vi "Build Waveform.vi"(6 "sampling config":cluster{"Fs":dbl, "#s":dbl}={"Fs"=1000.0, "#s"=1000.0} {"Fs" format="%.2p"}, 8 "error in (no error)":errorcluster, 11 "Config":T1={"Frequency"=10.0, "Voltage (V)"=1.0, "Signal type"=enum."Sine Wave", "Square wave duty cycle (%)"=50.0, "Offset (V)"=0.01, "DC shift"=FALSE} {"Square wave duty cycle (%)" format="%0.2f"}) -> (0 "error out":errorcluster, 3 "Waveform":waveform(dbl)(graph))   [LabVIEW 2019]
doc: "This example demonstrates how to acquire a continuous amount of data (Waveform) using the DAQ device's internal clock. It also shows how to synchronize two devices for different device families (E Series, S Series, M Series, X Series, DSA, and SC Express), to simultaneously acquire the data.\n\nFor instructions on how to connect your signals to the DAQ device, refer to your device documentation."
uses:
  <vilib>/measure/NI_MABase.lvlib
panel:
  # "Generate Waveform"
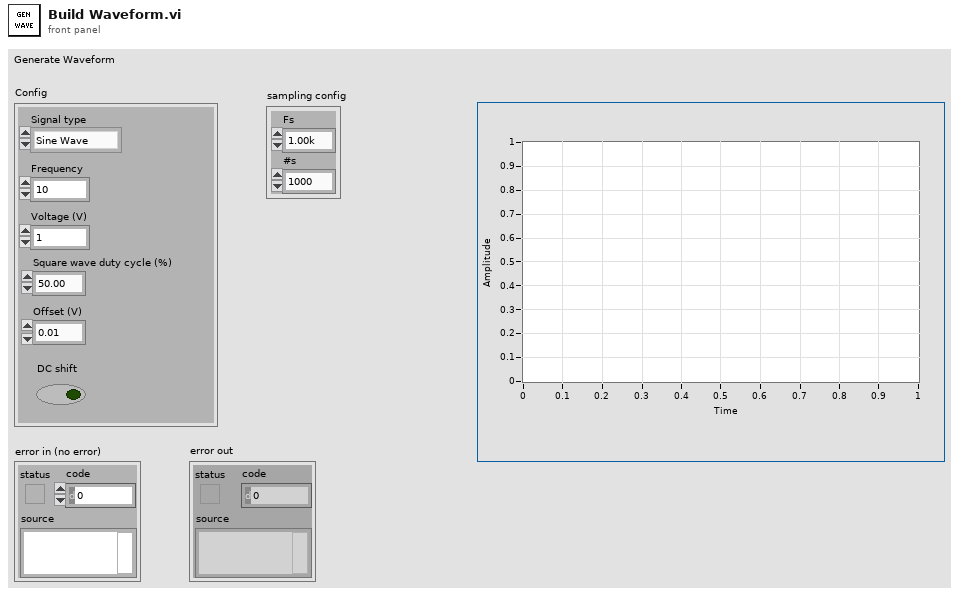
[diagram p1: front panel]
types:
  T1 = cluster{"Frequency":dbl, "Voltage (V)":dbl, "Signal type":enum16{"Sine Wave", "Triangle Wave", "Square Wave", "Sawtooth Wave"}, "Square wave duty cycle (%)":dbl, "Offset (V)":dbl, "DC shift":bool}
  T2 = enum16{"Sine Wave", "Triangle Wave", "Square Wave", "Sawtooth Wave"}
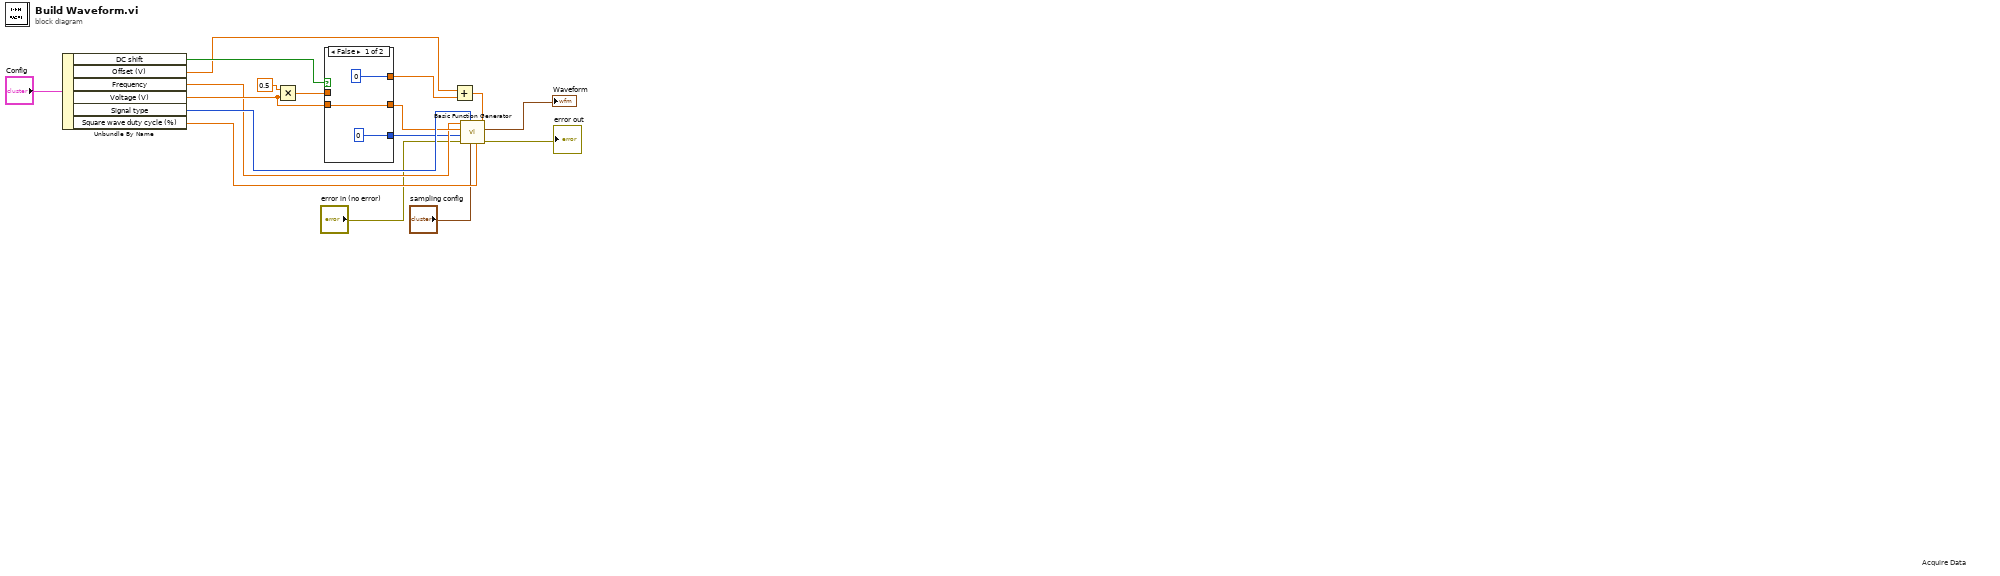
[diagram p0: block diagram]
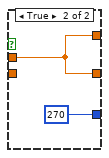
[diagram p2: hidden frame]
diagram:
  # "Acquire Data"
  n1 = Unbundle By Name("Config") -> ("DC shift"=w15:bool, "Offset (V)"=w14:dbl, "Frequency"=w6:dbl, "Voltage (V)"=w9:dbl, "Signal type"=w13:T2, "Square wave duty cycle (%)"=w4:dbl)
  n2 = Multiply(x=0.5, y=w9) -> (x*y=w11:dbl)
  n3 = case shown="False" w15 {
    tunnel: [0 w22] -> w10
    tunnel: w11 -> [_ w22]
    tunnel: [w19 w22] -> w7
    tunnel: w9 -> [w19 _]
    tunnel: [0 270] -> w5
    frame False {
    }
    frame True {
    }
  }
  n4 = Add(x=w14, y=w10) -> (x+y=w8:dbl)
  n5 = call <vilib>:"Basic Function Generator.vi"("offset"=w8, "square wave duty cycle (%)"=w4, "sampling info"="sampling config", "signal type"=w13, "error in (no error)"="error in (no error)", "phase"=w5, "amplitude"=w7, "frequency"=w6) -> ("error out"=→"error out":errorcluster, "signal out"=→"Waveform":waveform(dbl))  [unwired: 1 in, 1 out]
